vi "FSK_OBJ.vi"(7 "Mode":enum16{"Get", "Set"}(ring), 8 "error in":errorcluster, 11 "PROPERTIES IN":T1={"rate (bit/s)"=128.0, "bp (Bit Period)"=1e-06, "f1%"=80.0, "f2%"=20.0, "f1 (1 Freq)"=0.0, "f2 (0 Freq)"=0.0, "t (Time arry)"=[], "y1 (f1 cos arry)"=[], "y2 (f2 cos arry)"=[], "data length (B)"=3, "data size"=0, "sample size"=0.0} {"f2%" format="%#_6f"; "f1%" format="%#_6f"; "sample size" format="%#_13g"; "y2 (f2 cos arry)" format="%#_6f"; "y1 (f1 cos arry)" format="%#_6f"; "t (Time arry)" format="%#_6f"; "f2 (0 Freq)" format="%#_6f"; "f1 (1 Freq)" format="%#_6f"; "bp (Bit Period)" format="%#_13f"; "rate (bit/s)" format="%#_13g"}) -> (0 "error out":errorcluster, 3 "PROPERTIES OUT":T1={"rate (bit/s)"=128.0, "bp (Bit Period)"=1e-06, "f1%"=80.0, "f2%"=20.0, "f1 (1 Freq)"=0.0, "f2 (0 Freq)"=0.0, "t (Time arry)"=[], "y1 (f1 cos arry)"=[], "y2 (f2 cos arry)"=[], "data length (B)"=0, "data size"=0, "sample size"=0.0} {"f2%" format="%#_6f"; "f1%" format="%#_6f"; "sample size" format="%#_13g"; "y2 (f2 cos arry)" format="%#_6f"; "y1 (f1 cos arry)" format="%#_6f"; "t (Time arry)" format="%#_6f"; "f2 (0 Freq)" format="%#_6f"; "f1 (1 Freq)" format="%#_6f"; "bp (Bit Period)" format="%#_13f"; "rate (bit/s)" format="%#_13g"})   [LabVIEW 2013]
uses:
  FSK_OBJ - PROP.ctl
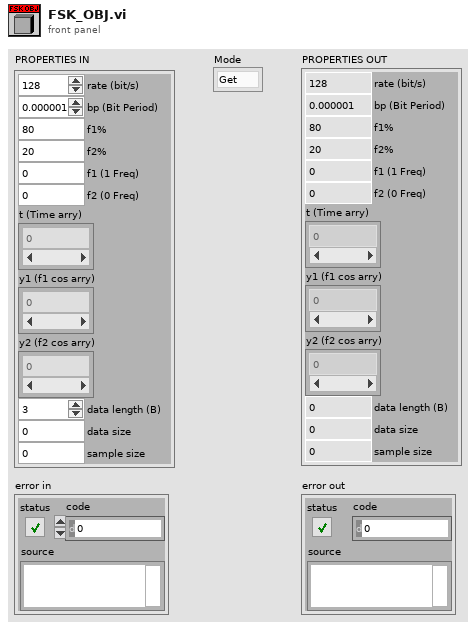
[diagram p1: front panel]
types:
  T1 = typedef "FSK_OBJ - PROP.ctl" = cluster{"rate (bit/s)":dbl, "bp (Bit Period)":dbl, "f1%":dbl, "f2%":dbl, "f1 (1 Freq)":dbl, "f2 (0 Freq)":dbl, "t (Time arry)":dbl[], "y1 (f1 cos arry)":dbl[], "y2 (f2 cos arry)":dbl[], "data length (B)":i32, "data size":i32, "sample size":dbl}
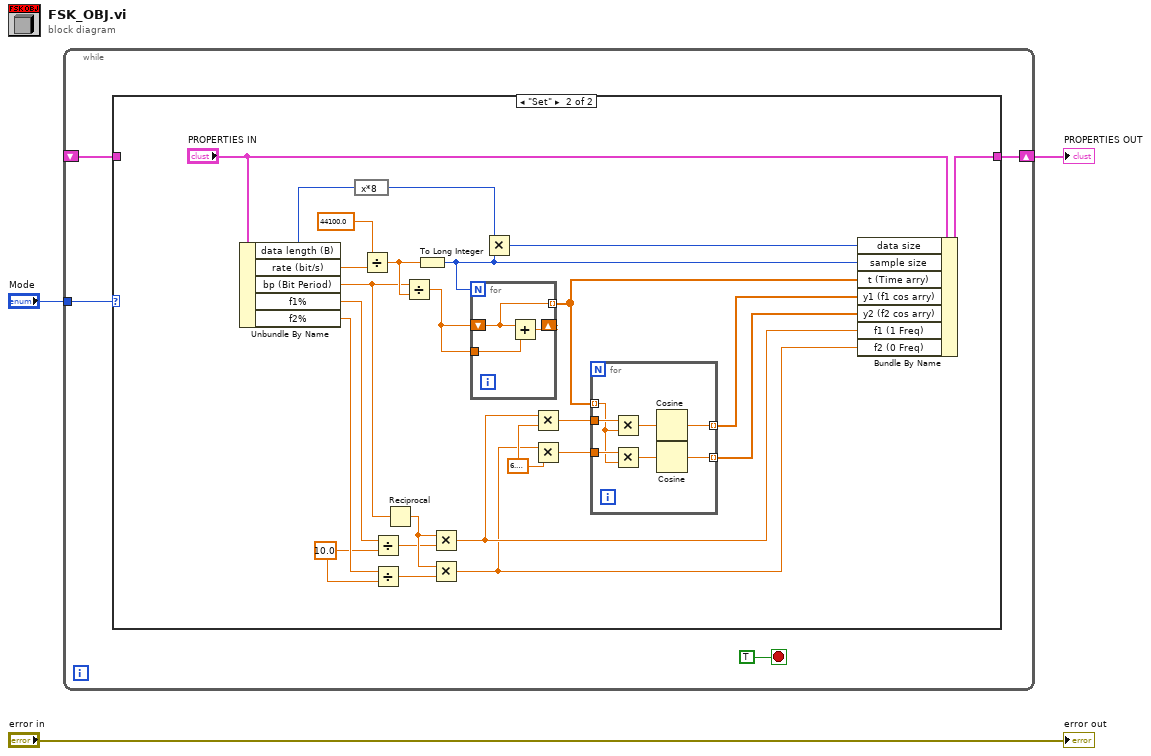
[diagram p0: block diagram]
diagram:
  n1 = while {
    tunnel: "Mode" -> [w6]
    shift-right: [w5] -> w2
    shift-left: _ -> [w4]
    stop <- TRUE stop-if-true
    n2 = case shown="\"Set\"" w6 {
      tunnel: [w8 w30] -> w5
      tunnel: w4 -> [w8 _]
      frame "Get", Default {
      }
      frame "Set" {
        w20 = 6.283185307179586
        w24 = 10.0 ("y")
        n3 = Unbundle By Name("PROPERTIES IN") -> ("data length (B)"=w12:i32, "rate (bit/s)"=w31:dbl, "bp (Bit Period)"=w28:dbl, "f1%"=w26:dbl, "f2%"=w25:dbl)
        n4 = expression code="x*8"(w12) -> (w11:i32)
        n5 = Divide(x=44100.0, y=w31) -> (x/y=w29:dbl)
        n6 = Divide(x=w26, y=w24) -> (x/y=w22:dbl)
        n7 = Divide(x=w25, y=w24) -> (x/y=w23:dbl)
        n8 = Reciprocal(x=w28) -> (1/x=w27:dbl)
        n9 = Divide(x=w28, y=w29) -> (x/y=w21:dbl)
        n10 = To Long Integer(number=w29) -> (32bit integer=w10:i32)
        n11 = Multiply(x=w27, y=w22) -> (x*y=w14:dbl)
        n12 = Multiply(x=w27, y=w23) -> (x*y=w13:dbl)
        n13 = for {
          N: w10 -> [_]
          shift-right: [w42] -> _
          shift-left: w21 -> [w41]
          tunnel: w21 -> [w43]
          tunnel: [w41] -> w17 mode=indexing
          n14 = Add(x=w41, y=w43) -> (x+y=w42:dbl)
        }
        n15 = Multiply(x=w11, y=w10) -> (x*y=w9:i32)
        n16 = Multiply(x=w14, y=w20) -> (x*y=w19:dbl)
        n17 = Multiply(x=w13, y=w20) -> (x*y=w18:dbl)
        n18 = for {
          tunnel: w19 -> [w39]
          tunnel: w18 -> [w40]
          tunnel: w17 -> [w38] mode=indexing
          tunnel: [w35] -> w16 mode=indexing
          tunnel: [w34] -> w15 mode=indexing
          n19 = Multiply(x=w39, y=w38) -> (x*y=w37:dbl)
          n20 = Multiply(x=w40, y=w38) -> (x*y=w36:dbl)
          n21 = Cosine(x=w37) -> (cos(x)=w35:dbl)
          n22 = Cosine(x=w36) -> (cos(x)=w34:dbl)
        }
        n23 = Bundle By Name(cluster="PROPERTIES IN", "data size"=w9, "sample size"=w10, "t (Time arry)"=w17, "y1 (f1 cos arry)"=w16, "y2 (f2 cos arry)"=w15, "f1 (1 Freq)"=w14, "f2 (0 Freq)"=w13) -> (w30:T1)
      }
    }
  }
  "PROPERTIES OUT" <- w2
  "error out" <- "error in"
